vi "Handle Command.vi"(8 "error in (no error)":errorcluster, 9 "Data":variant, 10 "Command":string, 11 "Inst.AH2500 in":refnum<class "Inst.AH2500.lvclass">) -> (0 "error out":errorcluster, 1 "Processed Data":variant, 2 "Command":string, 3 "Inst.AH2500 out":refnum<class "Inst.AH2500.lvclass">)   [LabVIEW 2019, in "Inst.AH2500.lvclass"]
uses:
  Inst.AH2500.lvclass
  <userlib>/LevyLab/Instrument Framework/Instrument Types/VSource/Instrument.VSource.lvclass
  Typedefs/Inst.AH2500.getAll--Cluster.ctl
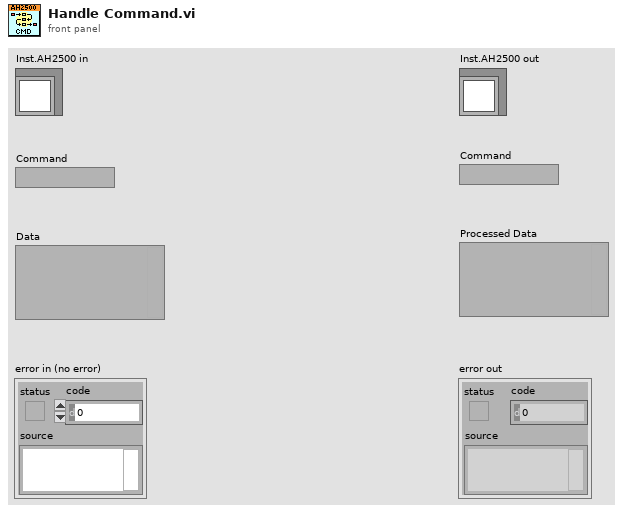
[diagram p1: front panel]
types:
  T1 = typedef "Inst.AH2500.lvclass/Inst.AH2500.getAll--Cluster.ctl" = cluster{"capacitance (pF)":dbl, "loss (nS)":dbl, "Vexc (V)":dbl}
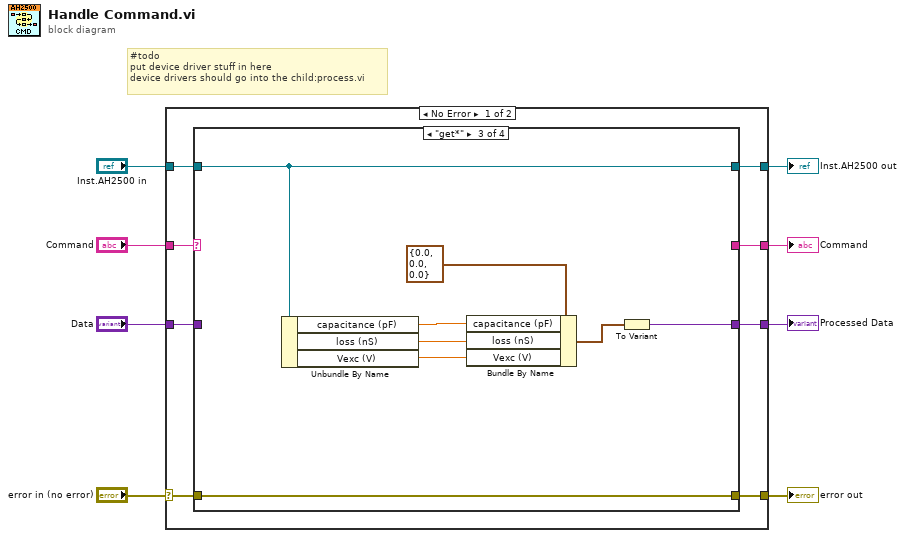
[diagram p0: block diagram]
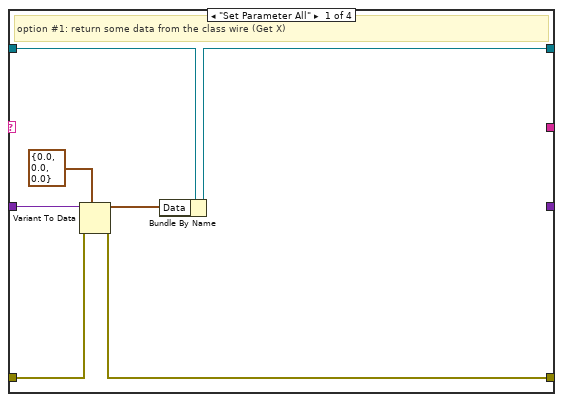
[diagram p2: hidden frame]
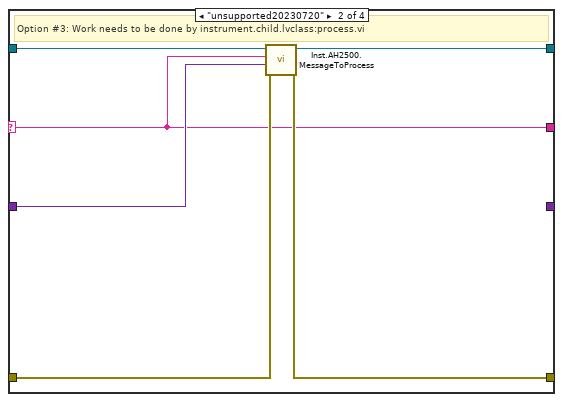
[diagram p3: hidden frame]
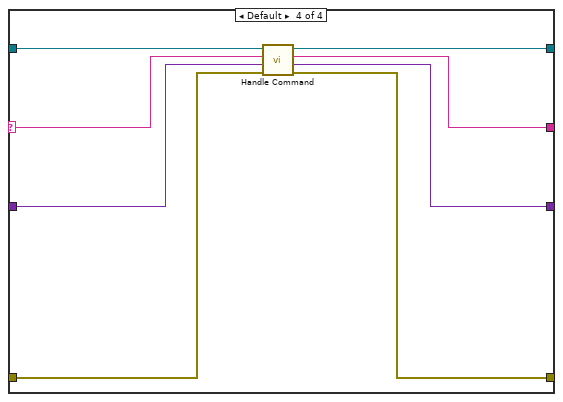
[diagram p4: hidden frame]
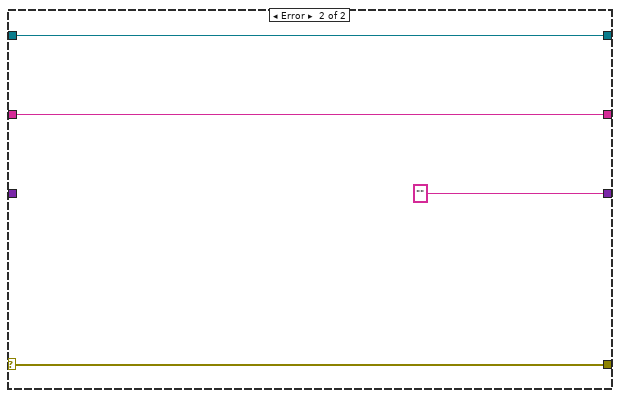
[diagram p5: hidden frame]
diagram:
  # "#todo\nput device driver stuff in here\ndevice drivers should go into the child:process.vi"
  n1 = case shown="No Error" "error in (no error)" {
    selector: "error in (no error)" -> [w10 w49]
    tunnel: [w12 w49] -> w6
    tunnel: [w14 w48] -> w5
    tunnel: "Inst.AH2500 in" -> [w15 w48]
    tunnel: "Command" -> [w16 w46]
    tunnel: [w13 "" ("String")] -> w3
    tunnel: "Data" -> [w9 _]
    tunnel: [w11 w46] -> w1
    frame No Error {
      n2 = case shown="\"get*\"" w16 {
        selector: w16 -> [_ w24 _ w39]
        tunnel: w15 -> [w17 w29 w37 w43]
        tunnel: [w18 w28 w37 w40] -> w14
        tunnel: [_ _ w36 w42] -> w13
        tunnel: w10 -> [w19 w27 w35 w44]
        tunnel: w9 -> [w23 w25 _ w45]
        tunnel: [w20 w26 w35 w41] -> w12
        tunnel: [_ w24 _ w38] -> w11
        frame "Set Parameter All" {
          # "option #1: return some data from the class wire (Get X)"
          n3 = Variant To Data(error in=w19, type=T1 {"capacitance (pF)"=0.0, "loss (nS)"=0.0, "Vexc (V)"=0.0} ("Data"), Variant=w23) -> (data=w22:T1, error out=w20:errorcluster)
          n4 = Bundle By Name(cluster=w17, "Data"=w22) -> (w18:refnum<class "Inst.AH2500.lvclass">)
        }
        frame "unsupported20230720" {
          # "Option #3: Work needs to be done by instrument.child.lvclass:process.vi"
          n5 = call "Inst.AH2500.MessageToProcess.vi"("error in (no error)"=w27, "Data"=w25, "Command"=w24, "Inst.AH2500 in"=w29) -> ("error out"=w26:errorcluster, "Inst.AH2500 out"=w28:refnum<class "Inst.AH2500.lvclass">)  [unwired: 6 in]
        }
        frame "get*" {
          n6 = Unbundle By Name(w37) -> ("capacitance (pF)"=w33:dbl, "loss (nS)"=w31:dbl, "Vexc (V)"=w30:dbl)
          n7 = Bundle By Name(cluster=T1 {"capacitance (pF)"=0.0, "loss (nS)"=0.0, "Vexc (V)"=0.0} ("getAll"), "capacitance (pF)"=w33, "loss (nS)"=w31, "Vexc (V)"=w30) -> (w32:T1)
          n8 = To Variant(anything=w32) -> (Variant=w36:variant)
        }
        frame Default {
          n9 = call-parent "Handle Command.vi"("error in (no error)"=w44, "Data"=w45, "Command"=w39, "Instrument in"=w43) -> ("error out"=w41:errorcluster, "Processed Data"=w42:variant, "Command"=w38:string, "Instrument out"=w40:refnum<class "Inst.AH2500.lvclass">)  [unwired: 4 in]
        }
      }
    }
    frame Error {
    }
  }
  "error out" <- w6
  "Inst.AH2500 out" <- w5
  "Command" <- w1
  "Processed Data" <- w3
